vi "Write ReceiveTimeOut.vi"(8 "error in (no error)":errorcluster, 10 "ReceiveTimeOut":i32=600, 11 "MelsecTCP in":refnum<class "MelsecMcNet.lvclass">) -> (0 "error out":errorcluster, 3 "MelsecTCP out":refnum<class "MelsecMcNet.lvclass">)   [LabVIEW 2020, in "MelsecMcNet.lvclass"]
uses:
  MelsecMcNet.lvclass
  MelsecMcNet.lvclass/MelsecMcNet.ctl
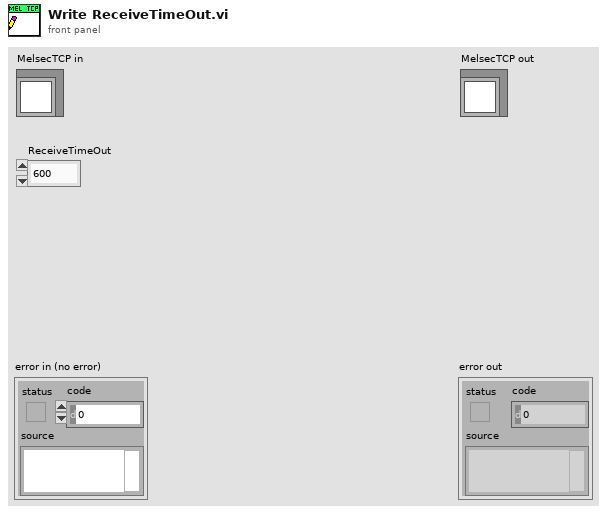
[diagram p1: front panel]
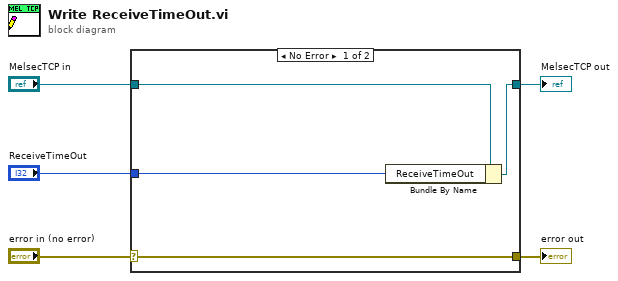
[diagram p0: block diagram]
diagram:
  n1 = case shown="No Error" "error in (no error)" {
    selector: "error in (no error)" -> [w9 w10]
    tunnel: [w9 w10] -> w4
    tunnel: [w7 w11] -> w2
    tunnel: "MelsecTCP in" -> [w8 w11]
    tunnel: "ReceiveTimeOut" -> [w6 _]
    frame No Error {
      n2 = Bundle By Name(cluster=w8, "ReceiveTimeOut"=w6) -> (w7:refnum<class "MelsecMcNet.lvclass">)
    }
    frame Error {
    }
  }
  "error out" <- w4
  "MelsecTCP out" <- w2
